vi "maquinadeestadosporeventos.vi"() -> ()   [LabVIEW 2016]
uses:
  Control 5.ctl
panel:
  in  "PARO":bool
  out "MD":bool
  out "MI":bool
  in  "S":bool
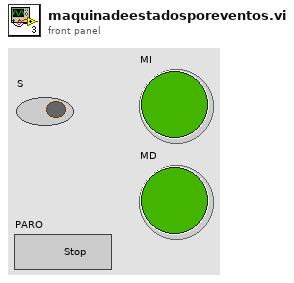
[diagram p1: front panel]
types:
  T1 = typedef "Control 5.ctl" = enum16{"avance", "espera", "izquierda", "derecha", "paro"}
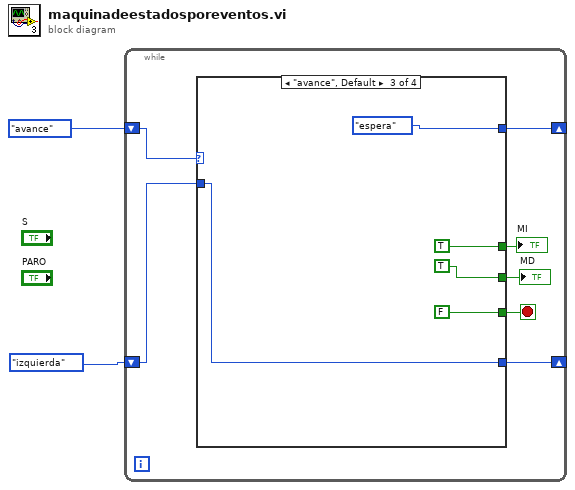
[diagram p0: block diagram]
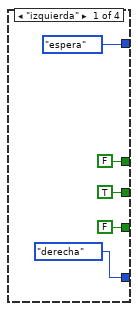
[diagram p2: hidden frame]
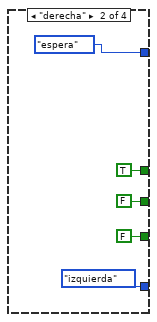
[diagram p3: hidden frame]
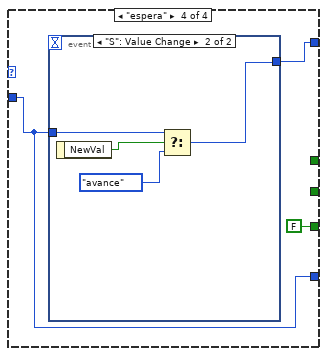
[diagram p4: hidden frame]
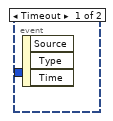
[diagram p5: hidden frame]
diagram:
  n1 = while {
    shift-right: [w6] -> _
    shift-left: Control_5."avance" -> [w4]
    shift-right: [w5] -> _
    shift-left: Control_5."izquierda" -> [w3]
    stop <- w7 stop-if-true
    n2 = case shown="\"avance\", Default" w4 {
      tunnel: [FALSE TRUE TRUE _] -> w9
      tunnel: [TRUE FALSE TRUE _] -> w8
      tunnel: [FALSE FALSE FALSE FALSE] -> w7
      tunnel: [Control_5."espera" Control_5."espera" Control_5."espera" w26] -> w6
      tunnel: [Control_5."derecha" Control_5."izquierda" w20 w25] -> w5
      tunnel: w3 -> [_ _ w20 w25]
      frame "izquierda" {
      }
      frame "derecha" {
      }
      frame "avance", Default {
      }
      frame "espera" {
        n3 = event shown="[1] \"S\": Value Change" {
          selector: _ -> [_ _]
          dyn-events: _ -> [_ _]
          timeout: _ -> [_ _]
          tunnel: [_ w29] -> w26
          tunnel: w25 -> [_ w28]
          event Timeout {
            n4 = event-data() -> ()  [unwired: 1 in, 3 out]
          }
          event "S": Value Change {
            n5 = event-data() -> ("NewVal"=w31:bool)  [unwired: 1 in]
            n6 = Select(t=w28, s=w31, f=Control_5."avance") -> (s? t:f=w29:T1)
          }
        }
      }
    }
    "MI" <- w9
    "MD" <- w8
  }
